vi "Create and Add Instruments.vi"(6 "Physical Intr CFGs":string[](array[string]), 7 "Target Enqueuer":refnum<class "Message Enqueuer.lvclass">, 8 "Error In":errorcluster, 11 "Host Measure and Stimulus Subsystems in":refnum<class "Host Measure and Stimulus Subsystems.lvclass">) -> (0 "Error Out":errorcluster, 3 "Host Measure and Stimulus Subsystems out":refnum<class "Host Measure and Stimulus Subsystems.lvclass">)   [LabVIEW 2023, in "HAL GOOP4.lvlib" / "Host Measure and Stimulus Subsystems.lvclass"]
uses:
  Host Measure and Stimulus Subsystems.lvclass
  <vilib>/ActorFramework/Message Enqueuer/Message Enqueuer.lvclass
  CFG Target/CFG Target.lvclass
  Configuration/Configuration JSON/Configuration JSON Base/CFG JSON.lvclass
  7b4e90f2-a286-44ae-9d63-d4d42d2d87e2.vi
  <vilib>/JDP Science/JSONtext/Find Item.vi
  <vilib>/JDP Science/JSONtext/Next JSON Value.vi
  <vilib>/JDP Science/JSONtext/String Subset.vi
  <vilib>/JDP Science/JSONtext/Parsing/Advance past next JSON Value (inlined COPY).vi
  <vilib>/JDP Science/JSONtext/Parsing/Advance past whitespace.vi
  <vilib>/JDP Science/JSONtext/Parsing/Advance past String.vi
  <vilib>/JDP Science/JSONtext/Parsing/Advance past Number.vi
  <vilib>/JDP Science/JSONtext/Parsing/Advance past Line Ending.vi
  <vilib>/JDP Science/JSONtext/Parsing/Parse Full Path or Item Name.vi
  <vilib>/JDP Science/JSONtext/Parsing/Advance past Array.vi
  <vilib>/JDP Science/JSONtext/Parsing/Advance past Object.vi
  <vilib>/JDP Science/JSONtext/support/Error Cluster From Code.vi
  <vilib>/JDP Science/JSONtext/Offset/Find Item Locations by Path.vi
  <vilib>/JDP Science/JSONtext/JSON text to Variant.vi
  <vilib>/Utility/error.llb/Error Cluster From Error Code.vi
  <vilib>/JDP Science/JSONtext/LVClass Serializer/JSONtext LVClass Serializer.lvclass
  <vilib>/ErrorRing/Error Ring.xnode
  Host Measure and Stimulus Subsystems.lvclass/Host Measure and Stimulus Subsystems.ctl
  Instrument/Instrument.lvclass
  D:/git/HAL/HAL GOOP4/Configuration/Configuration JSON/Configuration JSON Base/CFG JSON.lvclass
  D:/git/HAL/HAL GOOP4/Interfaces/IConfigure/IConfigure.lvclass
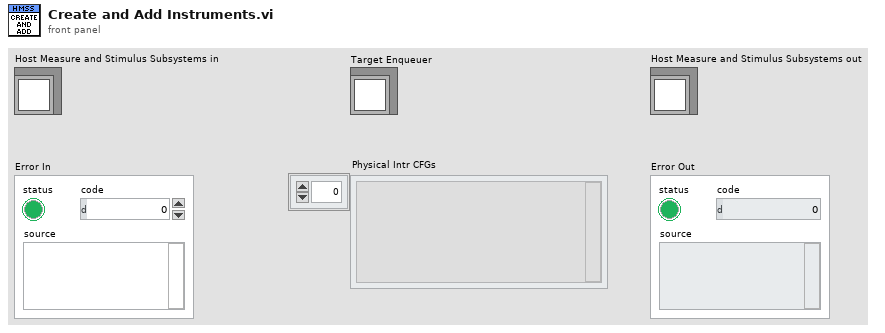
[diagram p1: front panel]
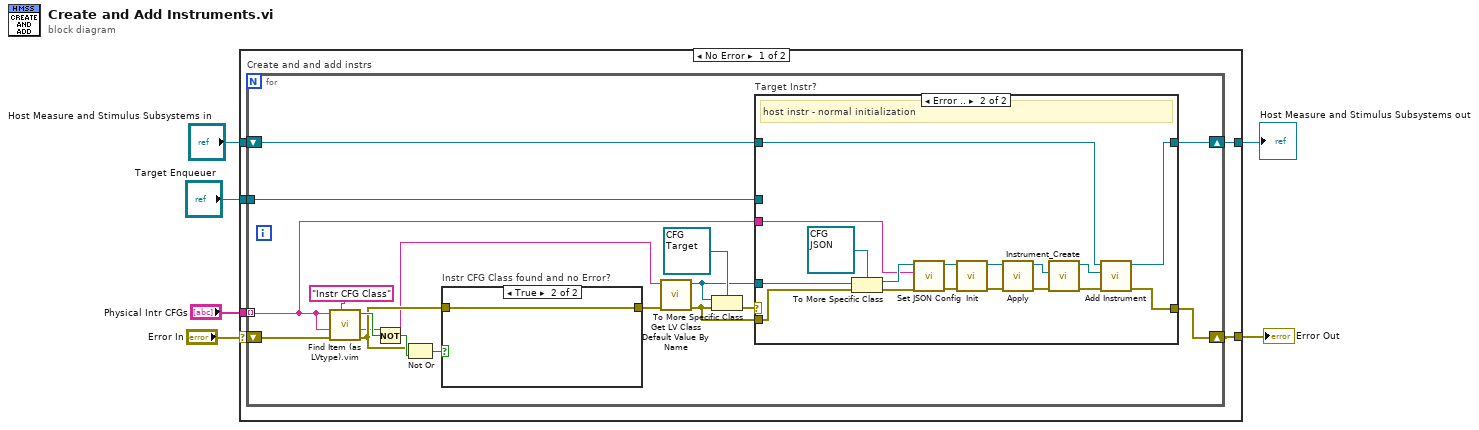
[diagram p0: block diagram]
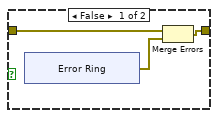
[diagram p3: hidden frame]
diagram:
  n1 = case shown="No Error" "Error In" {
    selector: "Error In" -> [w9 w58]
    tunnel: [w10 w58] -> w6
    tunnel: [w11 w59] -> w2
    tunnel: "Host Measure and Stimulus Subsystems in" -> [w12 w59]
    tunnel: "Physical Intr CFGs" -> [w8 _]
    tunnel: "Target Enqueuer" -> [w7 _]
    frame No Error {
      n2 = for "Create and and add instrs" {
        shift-right: [w20] -> w10
        shift-left: w9 -> [w21]
        tunnel: w8 -> [w18] mode=indexing
        shift-right: [w19] -> w11
        shift-left: w12 -> [w13]
        tunnel: w7 -> [w14]
        n3 = call "Find Item (as LVtype).vim"("$Path or Item Name"="Instr CFG Class", "error in (no error)"=w21, "Data Type and Default Value"=w18, "JSON"=w18) -> ("error out"=w25:errorcluster, "Data"=w23:string, "Found"=w27:bool)  [unwired: 4 in, 1 out]
        n4 = Not(x=w27) -> (.not. x?=w29:bool)
        n5 = Not Or(1:w29, 2:w25) -> (0:w28:bool)
        n6 = case "Instr CFG Class found and no Error?" shown="True" w28 {
          tunnel: [w51 w57] -> w26
          tunnel: w25 -> [w49 w57]
          frame False {
            n7 = xnode "Error Ring"() -> ("error out"=w50:errorcluster)
            n8 = Merge Errors(w49, w50) -> (w51:errorcluster)
          }
          frame True {
          }
        }
        n9 = call <vilib>:"Get LV Class Default Value By Name.vi"("error in (no error)"=w26, "class name"=w23) -> ("error out"=w16:errorcluster, "object"=w15:refnum<class>)  [unwired: 8 in]
        n10 = To More Specific Class(target class=refnum<class "CFG Target.lvclass"> refnum ("CFG Target.lvclass"), reference=w15, error in=w16) -> (error out=w17:errorcluster)  [unwired: 1 out]
        n11 = case "Target Instr?" shown="Error .." w17 {
          selector: w17 -> [w30 _]
          tunnel: [w30 w37] -> w20
          tunnel: w13 -> [w31 w36]
          tunnel: [w31 w35] -> w19
          tunnel: w18 -> [_ w34]
          tunnel: w16 -> [_ w33]
          tunnel: w15 -> [_ w32]
          tunnel: w14 -> [_ _]
          frame No Error {
            # "add instr to remote intrs map"
          }
          frame Error {
            # "host instr - normal initialization"
            n12 = To More Specific Class(target class=refnum<class "CFG JSON.lvclass"> refnum ("HAL GOOP4.lvlib:CFG JSON Base.lvclass"), reference=w32, error in=w33) -> (specific class reference=w45:refnum<class "CFG JSON.lvclass">, error out=w44:errorcluster)
            n13 = call "Set JSON Config.vi"("error in (no error)"=w44, "<JSON>Config>"=w34, "CFG Base in"=w45) -> ("error out"=w47:errorcluster, "CFG Base out"=w42:refnum<class "CFG JSON.lvclass">)  [unwired: 7 in]
            n14 = call-dynamic "Init.vi"("error in (no error)"=w47, "IConfigure in"=w42) -> ("error out"=w43:errorcluster, "IConfigure out"=w40:refnum<class "CFG JSON.lvclass">)  [unwired: 8 in]
            n15 = call-dynamic "Apply.vi"("error in (no error)"=w43, "IConfigure in"=w40) -> ("error out"=w41:errorcluster, "IConfigure out"=w39:refnum<class "CFG JSON.lvclass">)  [unwired: 8 in]
            n16 = call "Instrument_Create.vi"("Error In"=w41, "IConfigure"=w39) -> ("Error Out"=w48:errorcluster, "reference out"=w38:refnum<class "Instrument.lvclass">)  [unwired: 8 in]
            n17 = call "Add Instrument.vi"("error in"=w48, "Instrument"=w38, "Host Measure and Stimulus Subsystems in"=w36) -> ("error out"=w37:errorcluster, "Host Measure and Stimulus Subsystems out"=w35:refnum<class "Host Measure and Stimulus Subsystems.lvclass">)  [unwired: 7 in]
          }
        }
      }
    }
    frame Error {
    }
  }
  "Host Measure and Stimulus Subsystems out" <- w2
  "Error Out" <- w6
